vi "Write NET_HttpHeaders.vi"(8 "error in (no error)":errorcluster, 10 "NET_HttpHeaders":refnum<k24>, 11 "HTTPHeaders_NET in":refnum<class "HttpHeaders_NET.lvclass">) -> (0 "error out":errorcluster, 3 "HTTPHeaders_NET out":refnum<class "HttpHeaders_NET.lvclass">)   [LabVIEW 2018, in "LabVIEWHTTPClient_NET.lvlib" / "HttpHeaders_NET.lvclass"]
uses:
  HttpHeaders_NET.lvclass
  System.Net.Http
  HttpHeaders_NET.lvclass/HttpHeaders_NET.ctl
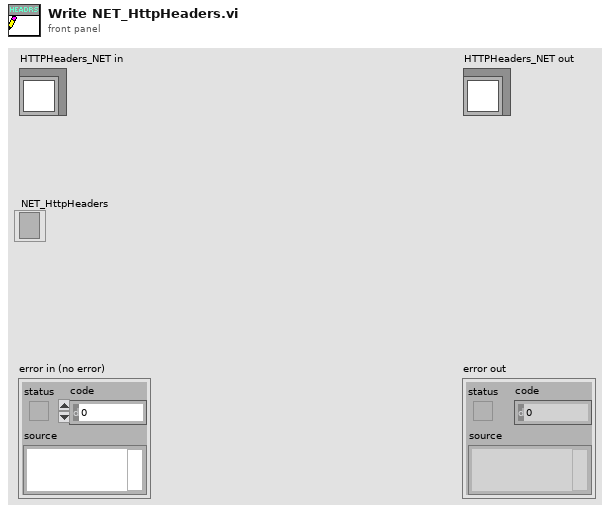
[diagram p1: front panel]
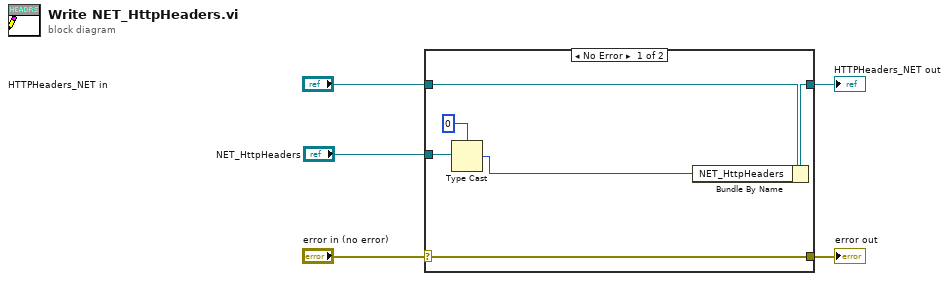
[diagram p0: block diagram]
diagram:
  n1 = case shown="No Error" "error in (no error)" {
    selector: "error in (no error)" -> [w11 w12]
    tunnel: [w11 w12] -> w4
    tunnel: [w9 w13] -> w2
    tunnel: "HTTPHeaders_NET in" -> [w10 w13]
    tunnel: "NET_HttpHeaders" -> [w8 _]
    frame No Error {
      n2 = Type Cast(type=i64 0 ("NET_HttpHeaders"), x=w8) -> (*(type *) &x=w6:i64)
      n3 = Bundle By Name(cluster=w10, "NET_HttpHeaders"=w6) -> (w9:refnum<class "HttpHeaders_NET.lvclass">)
    }
    frame Error {
    }
  }
  "error out" <- w4
  "HTTPHeaders_NET out" <- w2
